vi "Process data.vi"(8 "error in (no error)":errorcluster, 11 "processingTA in":refnum<class "processingTA.lvclass">) -> (0 "error out":errorcluster, 3 "processingTA out":refnum<class "processingTA.lvclass">)   [LabVIEW 2019, in "processingTA.lvlib" / "processingTA.lvclass"]
uses:
  processingTA.lvclass
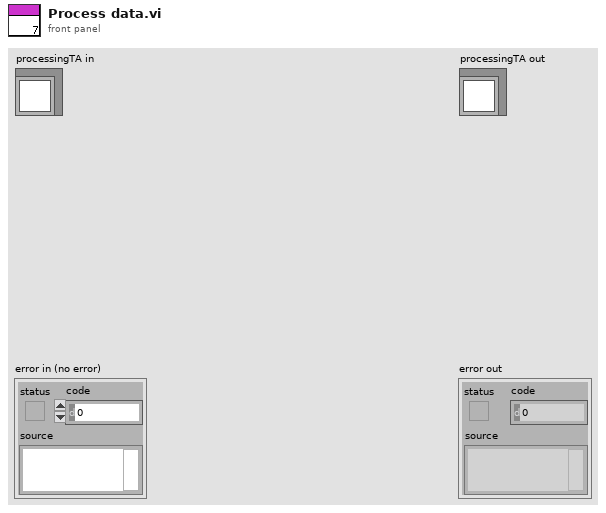
[diagram p1: front panel]
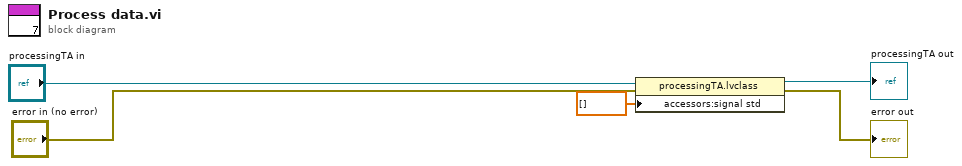
[diagram p0: block diagram]
diagram:
  n1 = property class="processingTA.lvclass"(reference="processingTA in", error in="error in (no error)", "accessors:signal std"=dbl[] [] ("signal std")) -> (reference out=→"processingTA out":refnum<class "processingTA.lvclass">, error out=→"error out":errorcluster)
